vi "Send Lights OFF.vi"(8 "error in":errorcluster) -> (0 "error out":errorcluster, 3 "Timeout?":bool)   [LabVIEW 2013]
uses:
  MsgQ Loops enum.ctl
  Main MsgQ.lvlib
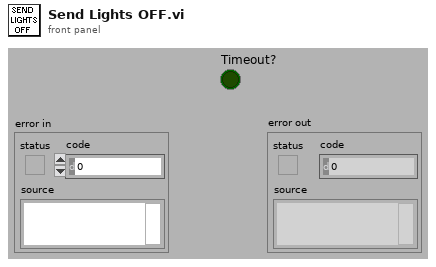
[diagram p1: front panel]
types:
  T1 = typedef "Main MsgQ.lvlib/MsgQ Loops enum.ctl" = enum16{"User Interface", "Image Acq"}
  T2 = typedef "Digital Output Lines cluster.ctl" = cluster{"Part Ready (0.0)":bool, "Part Status 0 (0.1)":bool, "Part Status 1 (0.2)":bool, "Part Status 2 (0.3)":bool, "Part Good (0.4)":bool, "Part Bad (0.5)":bool, "Defect (0.6)":bool, "Unused (0.7)":bool, "Unused (1.0)":bool, "Unused (1.1)":bool, "Unused (1.2)":bool, "Unused (1.3)":bool, "Unused (1.4)":bool, "Unused (1.5)":bool, "Unused (1.6)":bool, "Unused (1.7)":bool, "Unused (2.0)":bool, "Part Status 0 (2.1)":bool, "Part Status 1 (2.2)":bool, "Part Status 2 (2.3)":bool, "Part Good (2.4)":bool, "Part Bad (2.5)":bool, "Defect (2.6)":bool, "Unused (2.7)":bool, "Unused (3.0)":bool, "Unused (3.1)":bool, "Unused (3.2)":bool, "Unused (3.3)":bool, "Unused (3.4)":bool, "Unused (3.5)":bool, "Unused (3.6)":bool, "Unused (3.7)":bool}
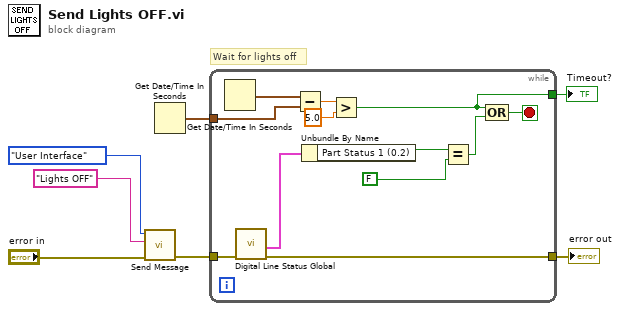
[diagram p0: block diagram]
diagram:
  # "Wait for lights off"
  n1 = call "Send Message.vi"("error in (no error)"="error in", "Message String"="Lights OFF", "Send to MsgQ"=MsgQ_Loops_enum."User Interface") -> ("error out"=w4:errorcluster)  [unwired: 1 in, 7 out]
  n2 = Get Date/Time In Seconds() -> (seconds since 1Jan1904=w3:timestamp)
  n3 = while {
    tunnel: w4 -> [w19]
    tunnel: w3 -> [w16]
    tunnel: [w8] -> w2
    tunnel: [w9] -> w1
    stop <- w10 stop-if-true
    n4 = Get Date/Time In Seconds() -> (seconds since 1Jan1904=w17:timestamp)
    n5 = call "Digital Line Status Global.vi"("error in"=w19) -> ("error out"=w9:errorcluster, "D0 Lines"=w18:T2)  [unwired: 3 in, 6 out]
    n6 = Subtract(x=w17, y=w16) -> (x-y=w15:dbl)
    n7 = Unbundle By Name(w18) -> ("Part Status 1 (0.2)"=w13:bool)
    n8 = Greater?(x=w15, y=5.0) -> (0:w8:bool)
    n9 = Equal?(x=w13, y=FALSE) -> (x = y?=w11:bool)
    n10 = Compound Arithmetic op=OR(w8, w11) -> (w10:bool)
  }
  "error out" <- w1
  "Timeout?" <- w2
